vi "Host.vi"() -> ()   [LabVIEW 2018]
uses:
  <instrlib>/niDCPower/nidcpower.llb/niDCPower Measurement Type.ctl
panel:
  in  "Период опроса, мс":u32=2000
  in  "ИОС":bool caption="ИОС вкл/выкл"
  out "ИОС_cur, A":dbl caption="measurement" format="%_6g"
  out "ИОС Chart":dbl(graph)=0.09491557293549348 caption="Waveform Chart 5"
  in  "ИОС, V":dbl=5.0 caption="voltage level" format="%_6p"
  in  "ИОС_curlim, A":dbl=0.1 caption="current limit" format="%_6p"
  in  "ИОС":refnum<k15>="PXI1Slot4" caption="instrument handle"
  in  "VRES_h_selcur":dbl=0.015 caption="current limit" format="%_6p"
  out "VRES_h":i32
  out "VRES_h":bool
  out "VRES_h_cur, A":dbl caption="measurement" format="%_6g"
  out "VRES_h Chart":dbl(graph)=-6.889343232631937
  in  "VRES_h, V":dbl=5.0 caption="voltage level" format="%_6p"
  in  "VRES_h_curlim, A":dbl=0.02 caption="current limit" format="%_6p"
  in  "Стоп":bool
  in  "Питание":bool
  in  "SEL_T, мс":u32=100
  in  "SIM_SEL":bool
  out "SEL":bool
  in  "VDD20_selcur":dbl=0.2 caption="current limit" format="%_6p"
  in  "VDD33_selcur":dbl=0.05 caption="current limit" format="%_6p"
  in  "VDDPIX_selcur":dbl=0.02 caption="current limit" format="%_6p"
  out "VDD20":i32
  out "VDD20":bool
  out "VDD33":i32
  out "VDD33":bool
  out "VDDPIX":i32
  out "VDDPIX":bool
  in  "VDD20, V":dbl=5.0 caption="voltage level" format="%_6p"
  in  "VDD20_curlim, A":dbl=0.4 caption="current limit" format="%_6p"
  in  "VDD33_curlim, A":dbl=0.1 caption="current limit" format="%_6p"
  out "VDD20_cur, A":dbl caption="measurement" format="%_6g"
  out "VDD33_cur, A":dbl caption="measurement" format="%_6g"
  in  "VDD33, V":dbl=5.0 caption="voltage level" format="%_6p"
  in  "VDDPIX, V":dbl=5.0 caption="voltage level" format="%_6p"
  in  "VDDPIX_curlim, A":dbl=0.05 caption="current limit" format="%_6p"
  out "VDDPIX_cur, A":dbl caption="measurement" format="%_6g"
  out "VDD33 Chart":dbl(graph)=0.0006520018718277456
  out "VDDPIX Chart":dbl(graph)=-6.889343232631937
  out "VDD20 Chart":dbl(graph)=0.09491557293549348 caption="Waveform Chart 5"
  in  "VDD20_VDD33":refnum<k15>="PXI1Slot2" caption="instrument handle"
  in  "VDDPIX_VRES_h":refnum<k15>="PXI1Slot3" caption="instrument handle"
  in  "SEL":path=path "C:/VPL/LabView_PRJ/CMV4000_22009/SEL"
  out "Номер образца":string="0"
  # "При испытаниях на лазере не забыть сделать особый опрос канала VDDPIX"
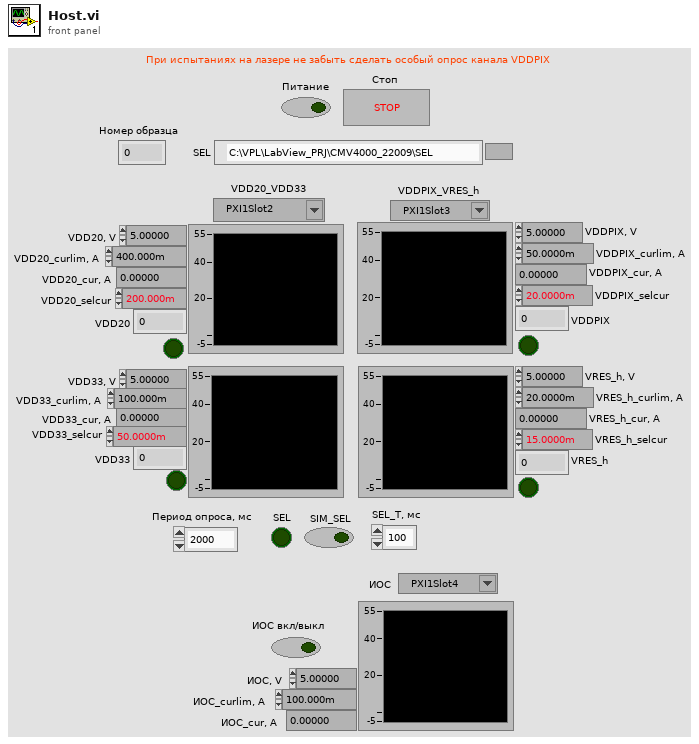
[diagram p1: front panel]
types:
  T1 = enum16{"open", "replace", "create", "open or create", "replace or create", "replace or create with confirmation"}
  T2 = typedef "niDCPower Measurement Type.ctl" = i32
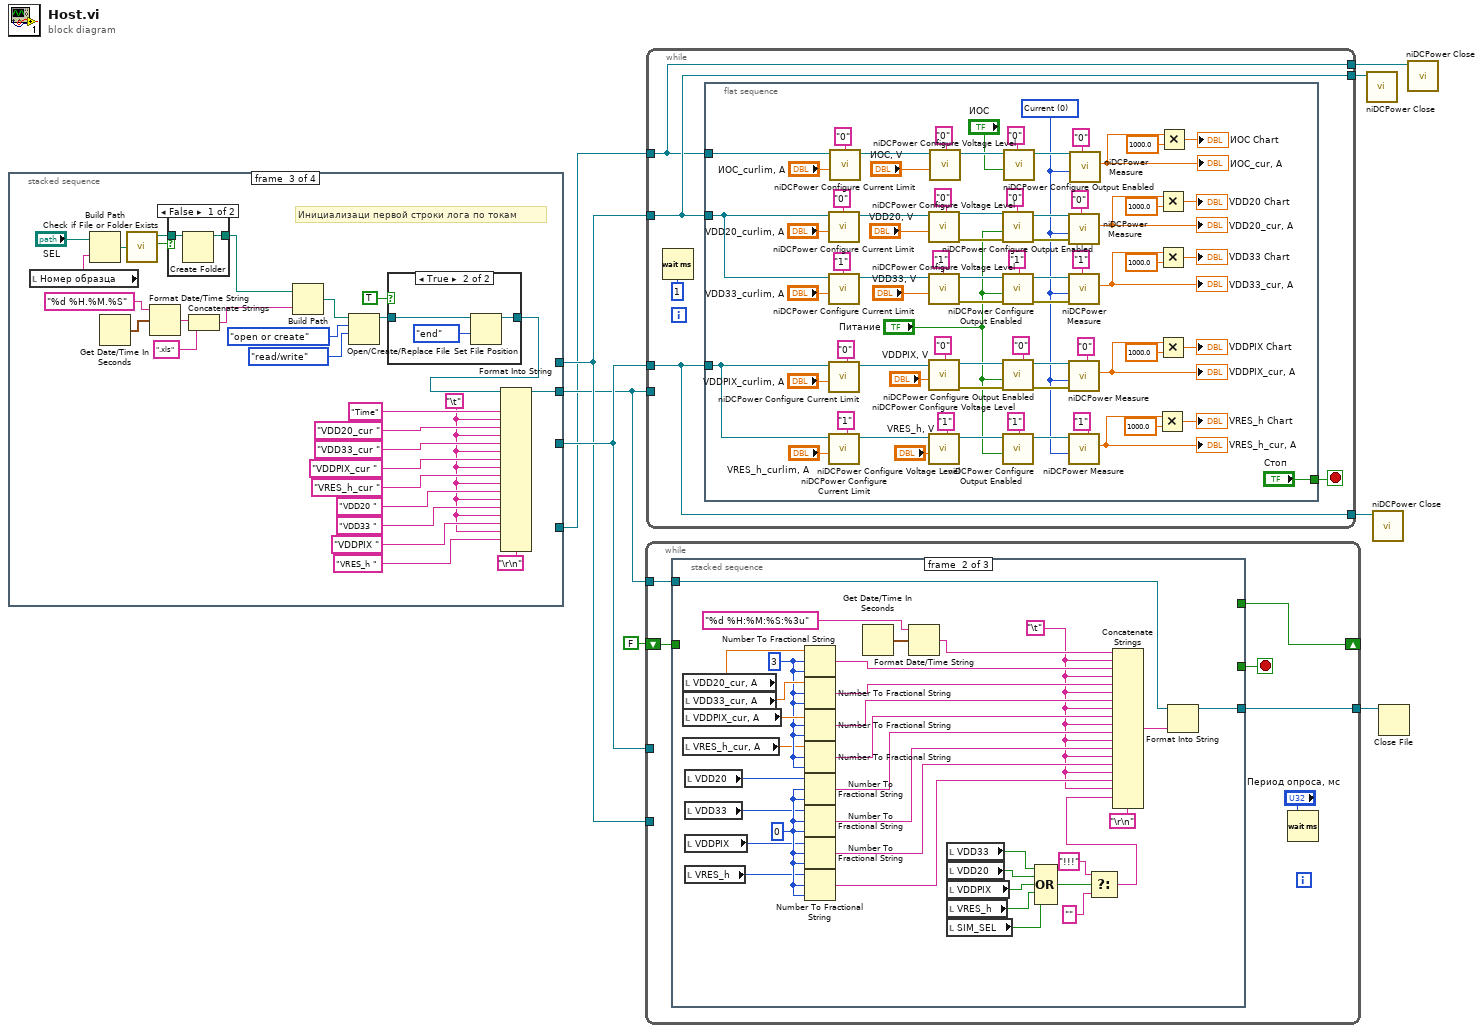
[diagram p0: block diagram]
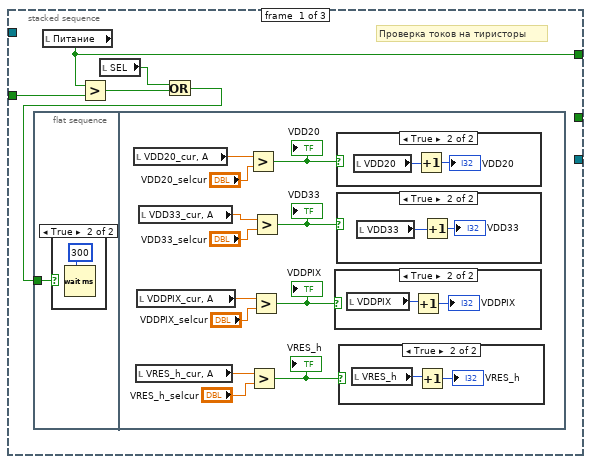
[diagram p2: hidden frame]
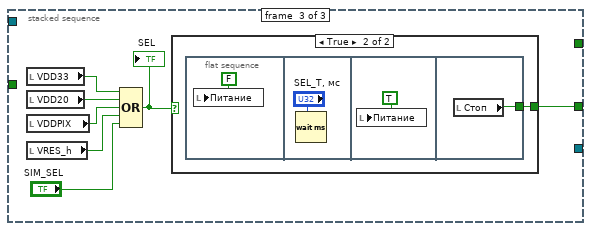
[diagram p8: hidden frame]
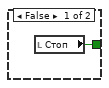
[diagram p9: hidden frame]
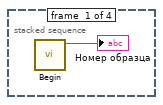
[diagram p10: hidden frame]
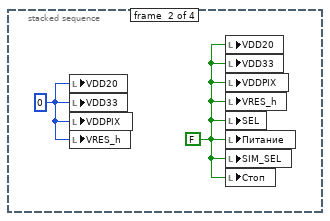
[diagram p11: hidden frame]
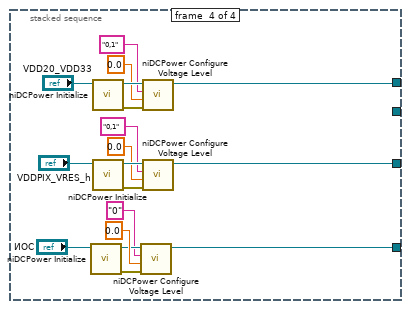
[diagram p14: hidden frame]
diagram:
  n1 = stacked-sequence {
    tunnel: [_ _ _ w56] -> w6
    tunnel: [_ _ _ w55] -> w5
    tunnel: [_ _ w25 _] -> w4
    tunnel: [_ _ _ w49] -> w2
    frame #0 {
      n2 = call "Begin.vi"() -> ("Номер образца 2"=→"Номер образца":string)  [unwired: 11 in]
    }
    frame #1 {
      w11 = 0
      w12 = FALSE
      n3 = local write "VDD20"(w11) -> ()
      n4 = local write "VDD33"(w11) -> ()
      n5 = local write "VDDPIX"(w11) -> ()
      n6 = local write "VRES_h"(w11) -> ()
      n7 = local write "VDD20"(w12) -> ()
      n8 = local write "VDD33"(w12) -> ()
      n9 = local write "VDDPIX"(w12) -> ()
      n10 = local write "VRES_h"(w12) -> ()
      n11 = local write "SEL"(w12) -> ()
      n12 = local write "Питание"(w12) -> ()
      n13 = local write "SIM_SEL"(w12) -> ()
      n14 = local write "Стоп"(w12) -> ()
    }
    frame #2 {
      w15 = "\t"
      # "Инициализаци первой строки лога по токам"
      n15 = local read "Номер образца"() -> (w37:string)
      n16 = Build Path(base path="SEL", name or relative path=w37) -> (appended path=w39:path)
      n17 = Get Date/Time In Seconds() -> (seconds since 1Jan1904=w32:timestamp)
      n18 = call <vilib>:"Check if File or Folder Exists.vi"("path"=w39) -> ("file or folder exists?"=w40:bool, "dup path"=w41:path)  [unwired: 8 in, 1 out]
      n19 = Format Date/Time String(time format string (%c)="%d %H.%M.%S", seconds (now)=w32) -> (date/time string=w29:string)  [unwired: 1 in]
      n20 = case shown="False" w40 {
        tunnel: w41 -> [w47 w48]
        tunnel: [w46 w48] -> w24
        frame False {
          n21 = Create Folder(path (use dialog)=w47) -> (created path=w46:path)  [unwired: 2 in, 2 out]
        }
        frame True {
        }
      }
      n22 = Concatenate Strings(w29, ".xls" ("string")) -> (w27:string)
      n23 = Build Path(base path=w24, name or relative path=w27) -> (appended path=w30:path)
      n24 = Open/Create/Replace File(file path (use dialog)=w30, operation (0:open)=T1."open or create", access (0:read/write)=enum16{"read/write", "read-only", "write-only"}."read/write") -> (refnum out=w33:refnum<file>)  [unwired: 3 in, 2 out]
      n25 = case shown="True" TRUE {
        tunnel: w33 -> [w42 w45]
        tunnel: [w42 w43] -> w26
        frame False {
        }
        frame True {
          n26 = Set File Position(refnum=w45, from (0:start)=enum16{"start", "end", "current"}."end") -> (refnum out=w43:refnum<file>)  [unwired: 2 in, 1 out]
        }
      }
      n27 = Format Into String(initial string=w26, "Time" ("input 1"), w15, "VDD20_cur " ("input 1"), w15, "VDD33_cur " ("input 1"), w15, "VDDPIX_cur " ("input 1"), w15, "VRES_h_cur " ("input 1"), w15, "VDD20 " ("input 1"), w15, "VDD33 " ("input 1"), w15, "VDDPIX " ("input 1"), w15, "VRES_h " ("input 1"), "\r\n") -> (resulting string=w25:refnum<file>)  [unwired: 2 in, 1 out]
    }
    frame #3 {
      n28 = call <instrlib>:"niDCPower Initialize.vi"("resource name"="ИОС") -> ("error out"=w52:errorcluster, "instrument handle out"=w51:refnum<k15>)  [unwired: 3 in, 6 out]
      n29 = call <instrlib>:"niDCPower Initialize.vi"("resource name"="VDD20_VDD33") -> ("error out"=w63:errorcluster, "instrument handle out"=w65:refnum<k15>)  [unwired: 3 in, 6 out]
      n30 = call <instrlib>:"niDCPower Initialize.vi"("resource name"="VDDPIX_VRES_h") -> ("error out"=w64:errorcluster, "instrument handle out"=w66:refnum<k15>)  [unwired: 3 in, 6 out]
      n31 = call <instrlib>:"niDCPower Configure Voltage Level.vi"("error in (no error)"=w52, "voltage level"=0.0, "channel name"="0", "instrument handle"=w51) -> ("instrument handle out"=w49:refnum<k15>)  [unwired: 6 in, 1 out]
      n32 = call <instrlib>:"niDCPower Configure Voltage Level.vi"("error in (no error)"=w63, "voltage level"=0.0, "channel name"="0,1", "instrument handle"=w65) -> ("instrument handle out"=w55:refnum<k15>)  [unwired: 6 in, 1 out]
      n33 = call <instrlib>:"niDCPower Configure Voltage Level.vi"("error in (no error)"=w64, "voltage level"=0.0, "channel name"="0,1", "instrument handle"=w66) -> ("instrument handle out"=w56:refnum<k15>)  [unwired: 6 in, 1 out]
    }
  }
  n34 = while {
    shift-right: [w72] -> _
    shift-left: FALSE -> [w71]
    tunnel: w4 -> [w70]
    tunnel: w6 -> [_]
    tunnel: w5 -> [_]
    tunnel: [w68] -> w3
    stop <- w69 stop-if-true
    n35 = stacked-sequence {
      tunnel: [w76 _ _] -> w72
      tunnel: w71 -> [w77 _ _]
      tunnel: w70 -> [_ w121 _]
      tunnel: [_ _ w137] -> w69
      tunnel: [_ w100 _] -> w68
      frame #0 {
        # "Проверка токов на тиристоры"
        n36 = flat-sequence {
          tunnel: w73 -> [w78]
          frame #0 {
            n37 = case shown="True" w78 {
              frame False {
              }
              frame True {
                n38 = Wait (ms)(milliseconds to wait=u32 300) -> ()  [unwired: 1 out]
              }
            }
          }
          frame #1 {
            n39 = local read "VDD20_cur, A"() -> (w85:dbl)
            n40 = local read "VRES_h_cur, A"() -> (w82:dbl)
            n41 = local read "VDDPIX_cur, A"() -> (w83:dbl)
            n42 = local read "VDD33_cur, A"() -> (w84:dbl)
            n43 = Greater?(x=w85, y="VDD20_selcur") -> (0:w90:bool)
            "VDD20" <- w90
            n44 = Greater?(x=w82, y="VRES_h_selcur") -> (0:w81:bool)
            "VRES_h" <- w81
            n45 = Greater?(x=w83, y="VDDPIX_selcur") -> (0:w86:bool)
            "VDDPIX" <- w86
            n46 = Greater?(x=w84, y="VDD33_selcur") -> (0:w88:bool)
            "VDD33" <- w88
            n47 = case shown="True" w86 {
              frame False {
              }
              frame True {
                n48 = local read "VDDPIX"() -> (w95:i32)
                n49 = Increment(x=w95) -> (x+1=→"VDDPIX":i32)
              }
            }
            n50 = case shown="True" w90 {
              frame False {
              }
              frame True {
                n51 = local read "VDD20"() -> (w99:i32)
                n52 = Increment(x=w99) -> (x+1=→"VDD20":i32)
              }
            }
            n53 = case shown="True" w88 {
              frame False {
              }
              frame True {
                n54 = local read "VDD33"() -> (w96:i32)
                n55 = Increment(x=w96) -> (x+1=→"VDD33":i32)
              }
            }
            n56 = case shown="True" w81 {
              frame False {
              }
              frame True {
                n57 = local read "VRES_h"() -> (w93:i32)
                n58 = Increment(x=w93) -> (x+1=→"VRES_h":i32)
              }
            }
          }
        }
        n59 = local read "Питание"() -> (w76:bool)
        n60 = Greater?(x=w76, y=w77) -> (0:w75:bool)
        n61 = local read "SEL"() -> (w74:bool)
        n62 = Or(x=w74, y=w75) -> (x .or. y?=w73:bool)
      }
      frame #1 {
        w114 = i16 0 ("width (-)")
        w113 = i16 3 ("width (-)")
        w105 = "\t"
        n63 = local read "VDD20_cur, A"() -> (w117:dbl)
        n64 = local read "VDD33_cur, A"() -> (w116:dbl)
        n65 = local read "VDDPIX_cur, A"() -> (w115:dbl)
        n66 = local read "VRES_h_cur, A"() -> (w112:dbl)
        n67 = local read "VDD20"() -> (w111:i32)
        n68 = local read "VDD33"() -> (w110:i32)
        n69 = local read "VDDPIX"() -> (w109:i32)
        n70 = local read "VRES_h"() -> (w108:i32)
        n71 = Number To Fractional String(number=w117, width (-)=w113, precision (6)=w113) -> (F-format string=w125:string)  [unwired: 1 in]
        n72 = Number To Fractional String(number=w116, width (-)=w113, precision (6)=w113) -> (F-format string=w124:string)  [unwired: 1 in]
        n73 = Number To Fractional String(number=w115, width (-)=w113, precision (6)=w113) -> (F-format string=w123:string)  [unwired: 1 in]
        n74 = Number To Fractional String(number=w112, width (-)=w113, precision (6)=w113) -> (F-format string=w120:string)  [unwired: 1 in]
        n75 = Number To Fractional String(number=w111, width (-)=w114, precision (6)=w114) -> (F-format string=w119:string)  [unwired: 1 in]
        n76 = Number To Fractional String(number=w110, width (-)=w114, precision (6)=w114) -> (F-format string=w118:string)  [unwired: 1 in]
        n77 = Number To Fractional String(number=w109, width (-)=w114, precision (6)=w114) -> (F-format string=w107:string)  [unwired: 1 in]
        n78 = Number To Fractional String(number=w108, width (-)=w114, precision (6)=w114) -> (F-format string=w106:string)  [unwired: 1 in]
        n79 = Get Date/Time In Seconds() -> (seconds since 1Jan1904=w134:timestamp)
        n80 = Format Date/Time String(time format string (%c)="%d %H:%M:%S:%3u", seconds (now)=w134) -> (date/time string=w126:string)  [unwired: 1 in]
        n81 = local read "VDD33"() -> (w129:bool)
        n82 = local read "VDD20"() -> (w128:bool)
        n83 = local read "VDDPIX"() -> (w127:bool)
        n84 = local read "VRES_h"() -> (w102:bool)
        n85 = local read "SIM_SEL"() -> (w101:bool)
        n86 = Compound Arithmetic op=OR(w129, w128, w127, w102, w101) -> (w122:bool)
        n87 = Select(t="!!!", s=w122, f="") -> (s? t:f=w104:string)
        n88 = Concatenate Strings(w126, w105, w125, w105, w124, w105, w123, w105, w120, w105, w119, w105, w118, w105, w107, w105, w106, w105, w104, "\r\n") -> (w133:string)
        n89 = Format Into String(initial string=w121, w133) -> (resulting string=w100:refnum<file>)  [unwired: 2 in, 1 out]
      }
      frame #2 {
        n90 = local read "VDD33"() -> (w141:bool)
        n91 = local read "VDD20"() -> (w140:bool)
        n92 = local read "VDDPIX"() -> (w139:bool)
        n93 = local read "VRES_h"() -> (w136:bool)
        n94 = Compound Arithmetic op=OR(w141, w140, w139, w136, "SIM_SEL") -> (w138:bool)
        "SEL" <- w138
        n95 = case shown="True" w138 {
          tunnel: [w142 w143] -> w137
          frame False {
            n96 = local read "Стоп"() -> (w142:bool)
          }
          frame True {
            n97 = flat-sequence {
              tunnel: [w147] -> w143
              frame #0 {
                n98 = local write "Питание"(FALSE ("SYS_RESET")) -> ()
              }
              frame #1 {
                n99 = Wait (ms)(milliseconds to wait="SEL_T, мс") -> ()  [unwired: 1 out]
              }
              frame #2 {
                n100 = local write "Питание"(TRUE ("SYS_RESET")) -> ()
              }
              frame #3 {
                n101 = local read "Стоп"() -> (w147:bool)
              }
            }
          }
        }
      }
    }
    n102 = Wait (ms)(milliseconds to wait="Период опроса, мс") -> ()  [unwired: 1 out]
  }
  n103 = while {
    tunnel: w6 -> [w150]
    tunnel: w5 -> [w151]
    tunnel: [w151] -> w9
    tunnel: [w150] -> w8
    tunnel: w4 -> [_]
    tunnel: w2 -> [w148]
    tunnel: [w148] -> w1
    stop <- w149 stop-if-true
    n104 = Wait (ms)(milliseconds to wait=u32 1) -> ()  [unwired: 1 out]
    n105 = flat-sequence {
      tunnel: w151 -> [w184]
      tunnel: w150 -> [w177]
      tunnel: ["Стоп"] -> w149
      tunnel: w148 -> [w165]
      frame #0 {
        w153 = T2 0 items=["Current", "Voltage"] ("measurement type")
        n106 = call <instrlib>:"niDCPower Configure Current Limit.vi"("current limit"="VDD20_curlim, A", "channel name"="0", "instrument handle"=w184) -> ("instrument handle out"=w215:refnum<k15>)  [unwired: 7 in, 1 out]
        n107 = call <instrlib>:"niDCPower Configure Current Limit.vi"("current limit"="VDD33_curlim, A", "channel name"="1", "instrument handle"=w184) -> ("instrument handle out"=w216:refnum<k15>)  [unwired: 7 in, 1 out]
        n108 = call <instrlib>:"niDCPower Configure Current Limit.vi"("current limit"="VDDPIX_curlim, A", "channel name"="0", "instrument handle"=w177) -> ("instrument handle out"=w198:refnum<k15>)  [unwired: 7 in, 1 out]
        n109 = call <instrlib>:"niDCPower Configure Current Limit.vi"("current limit"="VRES_h_curlim, A", "channel name"="1", "instrument handle"=w177) -> ("instrument handle out"=w175:refnum<k15>)  [unwired: 7 in, 1 out]
        n110 = call <instrlib>:"niDCPower Configure Current Limit.vi"("current limit"="ИОС_curlim, A", "channel name"="0", "instrument handle"=w165) -> ("instrument handle out"=w163:refnum<k15>)  [unwired: 7 in, 1 out]
        n111 = call <instrlib>:"niDCPower Configure Voltage Level.vi"("voltage level"="VDD20, V", "channel name"="0", "instrument handle"=w215) -> ("error out"=w208:errorcluster, "instrument handle out"=w211:refnum<k15>)  [unwired: 7 in]
        n112 = call <instrlib>:"niDCPower Configure Voltage Level.vi"("voltage level"="VDD33, V", "channel name"="1", "instrument handle"=w216) -> ("error out"=w209:errorcluster, "instrument handle out"=w210:refnum<k15>)  [unwired: 7 in]
        n113 = call <instrlib>:"niDCPower Configure Voltage Level.vi"("voltage level"="VDDPIX, V", "channel name"="0", "instrument handle"=w198) -> ("error out"=w202:errorcluster, "instrument handle out"=w203:refnum<k15>)  [unwired: 7 in]
        n114 = call <instrlib>:"niDCPower Configure Voltage Level.vi"("voltage level"="VRES_h, V", "channel name"="1", "instrument handle"=w175) -> ("instrument handle out"=w173:refnum<k15>)  [unwired: 7 in, 1 out]
        n115 = call <instrlib>:"niDCPower Configure Voltage Level.vi"("voltage level"="ИОС, V", "channel name"="0", "instrument handle"=w163) -> ("instrument handle out"=w161:refnum<k15>)  [unwired: 7 in, 1 out]
        n116 = call <instrlib>:"niDCPower Configure Output Enabled.vi"("error in (no error)"=w208, "output enabled"="Питание", "channel name"="0", "instrument handle"=w211) -> ("error out"=w220:errorcluster, "instrument handle out"=w219:refnum<k15>)  [unwired: 6 in]
        n117 = call <instrlib>:"niDCPower Configure Output Enabled.vi"("error in (no error)"=w209, "output enabled"="Питание", "channel name"="1", "instrument handle"=w210) -> ("error out"=w221:errorcluster, "instrument handle out"=w222:refnum<k15>)  [unwired: 6 in]
        n118 = call <instrlib>:"niDCPower Configure Output Enabled.vi"("error in (no error)"=w202, "output enabled"="Питание", "channel name"="0", "instrument handle"=w203) -> ("error out"=w194:errorcluster, "instrument handle out"=w195:refnum<k15>)  [unwired: 6 in]
        n119 = call <instrlib>:"niDCPower Configure Output Enabled.vi"("output enabled"="Питание", "channel name"="1", "instrument handle"=w173) -> ("instrument handle out"=w171:refnum<k15>)  [unwired: 7 in, 1 out]
        n120 = call <instrlib>:"niDCPower Configure Output Enabled.vi"("output enabled"="ИОС", "channel name"="0", "instrument handle"=w161) -> ("instrument handle out"=w159:refnum<k15>)  [unwired: 7 in, 1 out]
        n121 = call <instrlib>:"niDCPower Measure.vi"("error in (no error)"=w220, "measurement type"=w153, "channel name"="0", "instrument handle"=w219) -> ("measurement"=w187:dbl)  [unwired: 5 in, 2 out]
        "VDD20_cur, A" <- w187
        n122 = call <instrlib>:"niDCPower Measure.vi"("error in (no error)"=w221, "measurement type"=w153, "channel name"="1", "instrument handle"=w222) -> ("measurement"=w190:dbl)  [unwired: 5 in, 2 out]
        "VDD33_cur, A" <- w190
        n123 = call <instrlib>:"niDCPower Measure.vi"("error in (no error)"=w194, "measurement type"=w153, "channel name"="0", "instrument handle"=w195) -> ("measurement"=w188:dbl)  [unwired: 5 in, 2 out]
        "VDDPIX_cur, A" <- w188
        n124 = call <instrlib>:"niDCPower Measure.vi"("measurement type"=w153, "channel name"="1", "instrument handle"=w171) -> ("measurement"=w169:dbl)  [unwired: 6 in, 2 out]
        "VRES_h_cur, A" <- w169
        n125 = call <instrlib>:"niDCPower Measure.vi"("measurement type"=w153, "channel name"="0", "instrument handle"=w159) -> ("measurement"=w155:dbl)  [unwired: 6 in, 2 out]
        "ИОС_cur, A" <- w155
        n126 = Multiply(x=w169, y=1000.0) -> (x*y=→"VRES_h Chart":dbl)
        n127 = Multiply(x=w187, y=1000.0) -> (x*y=→"VDD20 Chart":dbl)
        n128 = Multiply(x=w190, y=1000.0) -> (x*y=→"VDD33 Chart":dbl)
        n129 = Multiply(x=w188, y=1000.0) -> (x*y=→"VDDPIX Chart":dbl)
        n130 = Multiply(x=w155, y=1000.0) -> (x*y=→"ИОС Chart":dbl)
      }
    }
  }
  n131 = call <instrlib>:"niDCPower Close.vi"("instrument handle"=w9) -> ()  [unwired: 10 in, 1 out]
  n132 = call <instrlib>:"niDCPower Close.vi"("instrument handle"=w8) -> ()  [unwired: 10 in, 1 out]
  n133 = Close File(refnum=w3) -> ()  [unwired: 1 in, 2 out]
  n134 = call <instrlib>:"niDCPower Close.vi"("instrument handle"=w1) -> ()  [unwired: 10 in, 1 out]
